vi "计算图像重排一维数组.vi"(1 "图像二维数组":dbl[][](array[numeric])) -> (0 "图像重排一维数组":dbl[](array[numeric]))   [LabVIEW 2018]
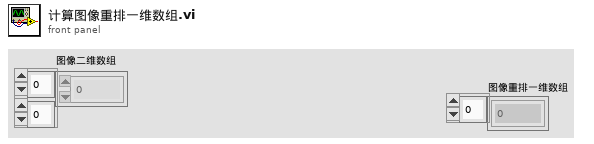
[diagram p1: front panel]
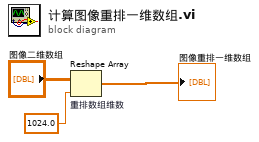
[diagram p0: block diagram]
diagram:
  n1 = Reshape Array "重排数组维数"("图像二维数组", 1024.0) -> (→"图像重排一维数组":dbl[])
